vi "Ignore Error.vi"(8 "error in":errorcluster, 9 "code":i32) -> (0 "error out":errorcluster)   [LabVIEW 2014, in "FTP.lvlib" / "FTP.lvclass"]
uses:
  FTP.lvclass
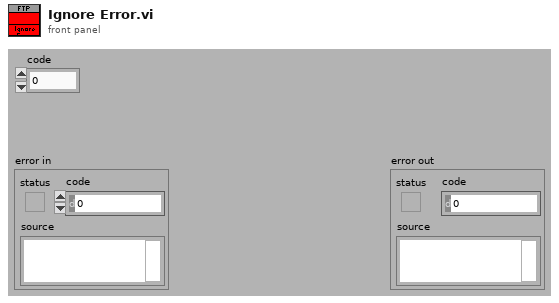
[diagram p1: front panel]
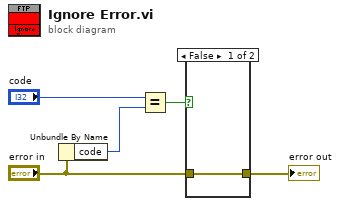
[diagram p0: block diagram]
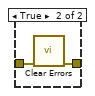
[diagram p2: hidden frame]
diagram:
  n1 = Unbundle By Name("error in") -> ("code"=w2:i32)
  n2 = Equal?(x="code", y=w2) -> (x = y?=w1:bool)
  n3 = case shown="False" w1 {
    tunnel: [w6 w8] -> w5
    tunnel: "error in" -> [w6 w7]
    frame False {
    }
    frame True {
      n4 = call <vilib>:"Clear Errors.vi"("error in (no error)"=w7) -> ("error out"=w8:errorcluster)  [unwired: 5 in, 1 out]
    }
  }
  "error out" <- w5
